vi "LED Test.vi"() -> ()   [LabVIEW 2018]
uses:
  <vilib>/Utility/RT CPU Load.ctl
  <vilib>/NI_Real-Time Target Support.lvlib
panel:
  in  "stop":bool
  out "CPU loads":T1[](array[typedef]) {"ISR (%)" format="%#.2f"; "Idle (%)" format="%#.2f"; "Background (%)" format="%#.2f"; "Normal (%)" format="%#.2f"; "Above Normal (%)" format="%#.2f"; "High (%)" format="%#.2g"; "Timed Structures (%)" format="%#.2g"; "Time Critical (%)" format="%#.2g"; "Total (%)" format="%#.2g"}
  out "error out":errorcluster
  in  "State":i32 min=0 max=3 step=1
  in  "LED Num":i32
  # "LED State.\n0\t----->Turns off the LED\n1\t----->Sets the LED to the device default color1\n2\t----->Sets the LED to the device default color2 (if available)\n3\t----->Toggle between off and default color1"
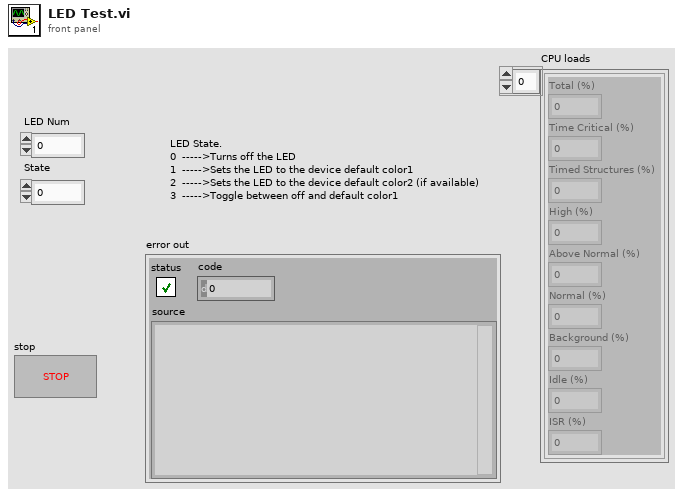
[diagram p1: front panel]
types:
  T1 = typedef "NI_Real-Time Target Support.lvlib/RT CPU Load.ctl" = cluster{"Total (%)":dbl, "Time Critical (%)":dbl, "Timed Structures (%)":dbl, "High (%)":dbl, "Above Normal (%)":dbl, "Normal (%)":dbl, "Background (%)":dbl, "Idle (%)":dbl, "ISR (%)":dbl}
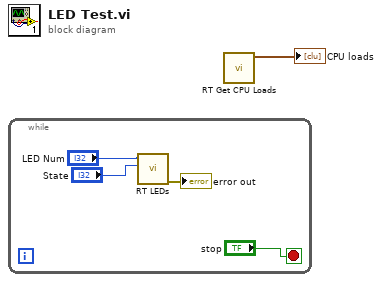
[diagram p0: block diagram]
diagram:
  n1 = while {
    stop <- "stop" stop-if-true
    n2 = call <vilib>:"RT LEDs.vi"("State"="State", "LED Num"="LED Num") -> ("error out"=→"error out":errorcluster)  [unwired: 4 in, 1 out]
  }
  n3 = call <vilib>:"RT Get CPU Loads.vi"() -> ("CPU loads"=→"CPU loads":T1[])  [unwired: 10 in, 1 out]
